vi "LWXPS_PositionerCorrectorDualSet.vi"(0 "Proportional gain":dbl, 1 "Integral gain":dbl, 2 "Derivative gain":dbl, 3 "Integration time":dbl, 4 "Derivative filter cut off frequency":dbl, 5 "Acceleration feedforward gain":dbl, 6 "Closed Loop Status":bool, 7 "Jerk feedforward gain":dbl, 8 "Positioner Name":string, 9 "Anti wind up time":dbl, 10 "XPS Reference IN":refnum<k24>, 11 "LabVIEW error IN":errorcluster) -> (14 "XPS Reference OUT":refnum<k24>, 15 "Returned error code":i32, 18 "XPS Error String":string, 19 "LabVIEW error OUT":errorcluster)   [LabVIEW 2014]
uses:
  D:/XPSQ8_LabView_Library/Development/Source/Dll/Newport.XPS.CommandInterface.dll
  Dll/Newport.XPS.CommandInterface.dll
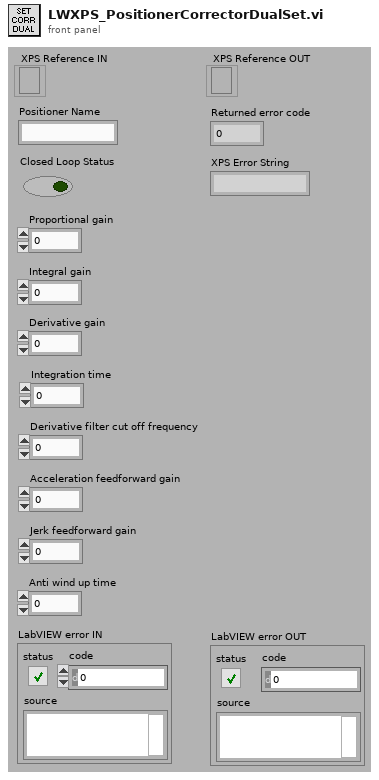
[diagram p1: front panel]
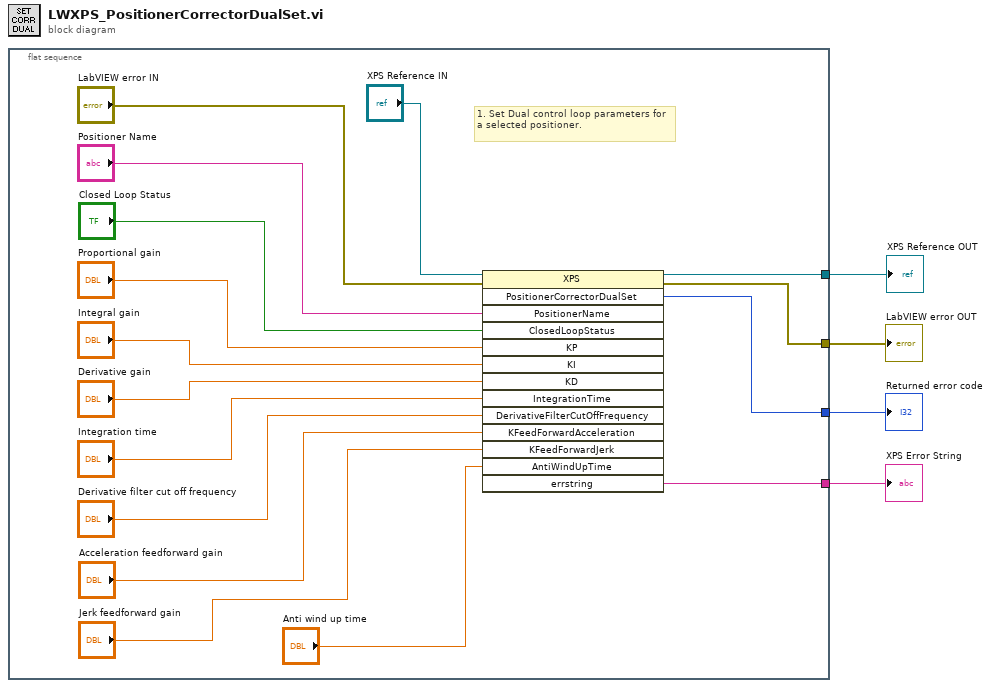
[diagram p0: block diagram]
diagram:
  n1 = flat-sequence {
    tunnel: [w16] -> w4
    tunnel: [w19] -> w3
    tunnel: [w18] -> w2
    tunnel: [w7] -> w1
    frame #0 {
      # "1. Set Dual control loop parameters for a selected positioner."
      n2 = invoke class="XPS" method="PositionerCorrectorDualSet"(reference="XPS Reference IN", error in="LabVIEW error IN", "PositionerName"="Positioner Name", "ClosedLoopStatus"="Closed Loop Status", "KP"="Proportional gain", "KI"="Integral gain", "KD"="Derivative gain", "IntegrationTime"="Integration time", "DerivativeFilterCutOffFrequency"="Derivative filter cut off frequency", "KFeedForwardAcceleration"="Acceleration feedforward gain", "KFeedForwardJerk"="Jerk feedforward gain", "AntiWindUpTime"="Anti wind up time") -> (reference out=w16:refnum<k24>, error out=w19:errorcluster, "PositionerCorrectorDualSet"=w18:i32, "errstring"=w7:string)  [unwired: 2 in, 10 out]
    }
  }
  "XPS Error String" <- w1
  "XPS Reference OUT" <- w4
  "LabVIEW error OUT" <- w3
  "Returned error code" <- w2
